vi "filter-designer.vi"() -> ()   [LabVIEW 2014]
uses:
  <vilib>/addons/Digital Filter Design/_Objects.llb/DFD Phase Setting.ctl
  <vilib>/addons/Digital Filter Design/Analysis.llb/DFD Plot Freq Response (Log-Spaced).vi
  <vilib>/addons/Digital Filter Design/NI_DigFilterLicensed.lvlib
panel:
  out "magnitude response":cluster{"bins":dbl[], "response FXP":dbl[]}[](graph)
  out "phase response":cluster{"bins":dbl[], "response FXP":dbl[]}[](graph)
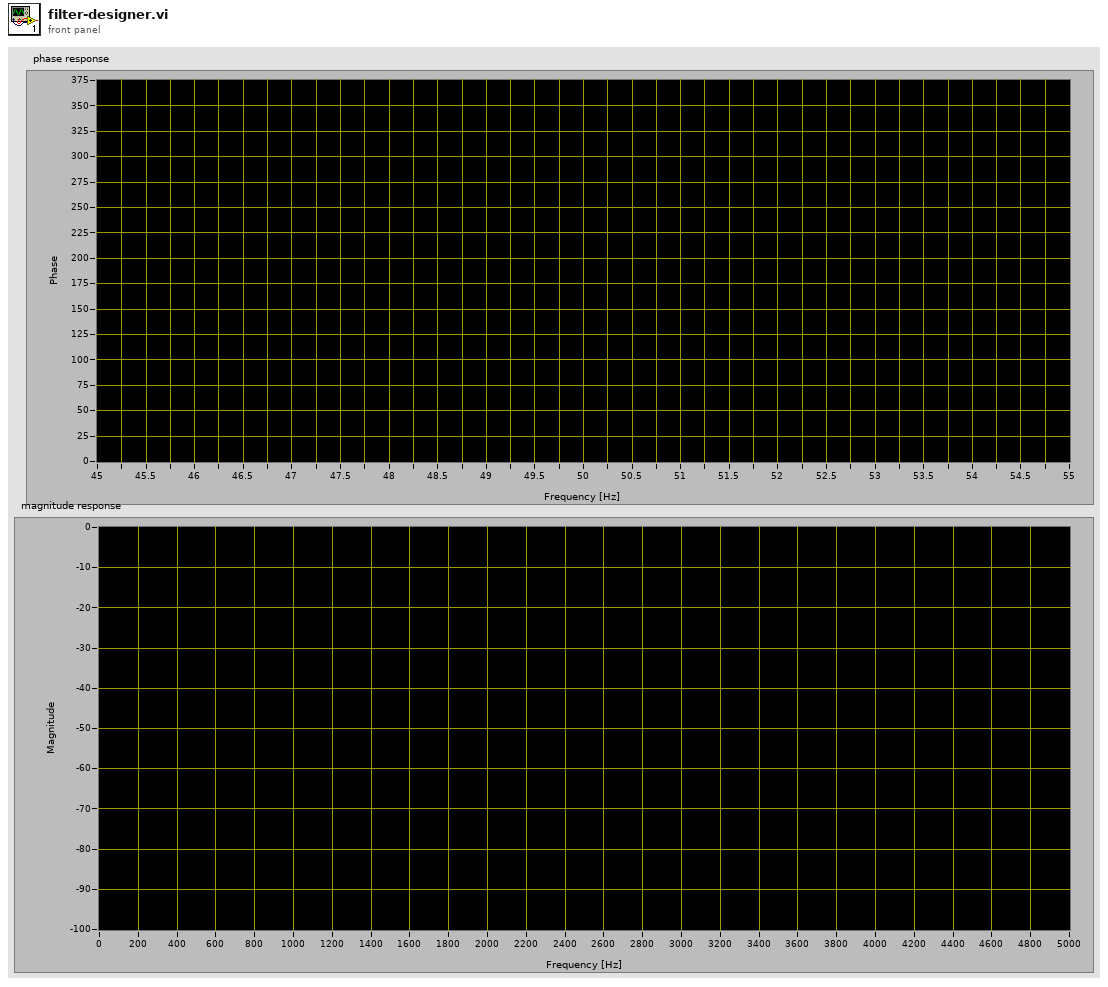
[diagram p1: front panel]
types:
  T1 = enum16{"Lowpass", "Highpass", "Bandpass", "Bandstop"}
  T2 = typedef "NI_DigFilterLicensed.lvlib/DFD Phase Setting.ctl" = cluster{"unwrap? (F)":bool, "degree? (F)":bool}
  T3 = typedef "NI_DigFilterLicensed.lvlib/DFD Filter Obj.ctl" = cluster{"mSRate_Fs":dbl, "mSRate_Version":string, "mSRate_Comments":string, "mSRate_OrgCoef":T4, "mSRate_CurCoef":T4, "mSRate_Quantized?":bool, "mSRate_QCoef":T4, "mSRate_QSettings":T6[], "mSRate_Order":i32, "mSRate_Scaling":cluster{"mSRate_ScaleByPowerOf2?":bool, "mSRate_ScaleType":T8}}
  T4 = typedef "NI_DigFilterLicensed.lvlib/DFD Filter Coef.ctl" = cluster{"type":T5, "gain":dbl, "coef a (k)":dbl[], "coef b (v)":dbl[]}
  T5 = typedef "NI_DigFilterLicensed.lvlib/DFD Filter Structure Type Selector.ctl" = enum16{"Undefined", "FIR Direct Form", "FIR Direct Form Transposed", "FIR Symmetric", "FIR Antisymmetric", "IIR Direct Form I", "IIR Direct Form I Transposed", "IIR Direct Form II", "IIR Direct Form II Transposed", "IIR Cascaded Second Order Sections Form I", "IIR Cascaded Second Order Sections Form I Transposed", "IIR Cascaded Second Order Sections Form II", "IIR Cascaded Second Order Sections Form II Transposed", "Lattice Allpass (basic sections)", "Lattice Allpass (one multiplier sections)", "Lattice Allpass (normalized sections)", "Lattice AR (basic sections)", "Lattice AR (one multiplier sections)", "Lattice AR (normalized sections)", "Lattice MA (minimum phase)", "Lattice MA (maximum phase)", "Lattice ARMA (basic sections)", "Lattice ARMA (one multiplier sections)", "Lattice ARMA (normalized sections)"}
  T6 = typedef "NI_DigFilterLicensed.lvlib/dfd_Internal Quantization Settings.ctl" = cluster{"source":T7, "wl":i16, "iwl":i16, "overflow mode":enum16{"Saturation", "Wrap"}, "rounding mode":enum16{"Nearest", "Truncation"}, "signed?":bool}
  T7 = typedef "NI_DigFilterLicensed.lvlib/dfd_Internal Quantization Srcs.ctl" = u16
  T8 = typedef "NI_DigFilterLicensed.lvlib/DFD Coef Norm Type.ctl" = enum16{"No Norm", "Time Domain 1-Norm", "Time Domain 2-Norm", "Time Domain Inf-Norm"}
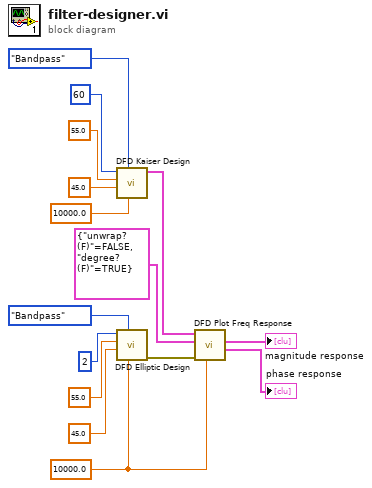
[diagram p0: block diagram]
diagram:
  w8 = 10000.0 ("fs [Hz]")
  n1 = call <vilib>:"DFD Kaiser Design.vi"("fs [Hz]"=10000.0, "filter type"=T1."Bandpass", "low cutoff freq [Hz]"=45.0, "high cutoff freq [Hz]"=55.0, "order"=60) -> ("filter out"=w1:T3)  [unwired: 5 in, 1 out]
  n2 = call <vilib>:"DFD Elliptic Design.vi"("fs [Hz]"=w8, "filter type"=T1."Bandpass", "low cutoff freq [Hz]"=45.0, "high cutoff freq [Hz]"=55.0, "order"=2) -> ("error out"=w11:errorcluster)  [unwired: 5 in, 1 out]
  n3 = call-poly <vilib>:"DFD Plot Freq Response.vi"("fs [Hz]"=w8, "error in (no error)"=w11, "phase view"=T2 {"unwrap? (F)"=FALSE, "degree? (F)"=TRUE}, "filter in"=w1) -> ("phase response"=→"phase response":cluster{"bins":dbl[], "response FXP":dbl[]}[], "magnitude response"=→"magnitude response":cluster{"bins":dbl[], "response FXP":dbl[]}[])  [unwired: 4 in, 2 out]
